vi "startNewLog.vi"(8 "error in (no error)":errorcluster, 11 "Logger in":refnum<class "Logger.lvclass">) -> (0 "error out":errorcluster, 3 "Logger out":refnum<class "Logger.lvclass">)   [LabVIEW 2013, in "Logger.lvclass"]
uses:
  Logger.lvclass
  Logger.lvclass/Logger.ctl
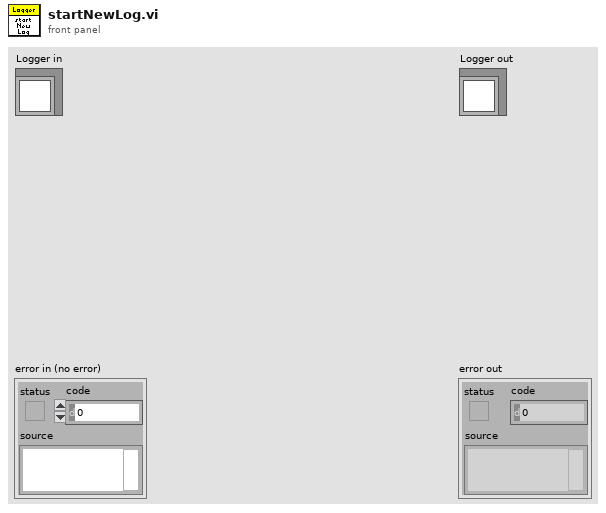
[diagram p1: front panel]
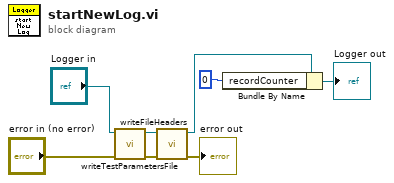
[diagram p0: block diagram]
diagram:
  n1 = call "writeTestParametersFile.vi"("error in (no error)"="error in (no error)", "Logger in"="Logger in") -> ("error out"=w1:errorcluster, "Logger out"=w3:refnum<class "Logger.lvclass">)  [unwired: 8 in]
  n2 = call "writeFileHeaders.vi"("error in (no error)"=w1, "Logger in"=w3) -> ("error out"=→"error out":errorcluster, "Logger out"=w7:refnum<class "Logger.lvclass">)  [unwired: 8 in]
  n3 = Bundle By Name(cluster=w7, "recordCounter"=u32 0) -> (→"Logger out":refnum<class "Logger.lvclass">)
